vi "Read Sondenmodell.Zustandsgrössen.vi"(8 "error in (no error)":errorcluster, 11 "Sondenmodell in":refnum<class "Sondenmodell.lvclass">) -> (0 "error out":errorcluster, 2 "Sondenmodell.Zustandsgrössen":T1, 3 "Sondenmodell out":refnum<class "Sondenmodell.lvclass">)   [LabVIEW 2016, in "Sondenmodell.lvclass"]
uses:
  Sondenmodell.lvclass
  Sondenmodell.lvclass/Sondenmodell.ctl
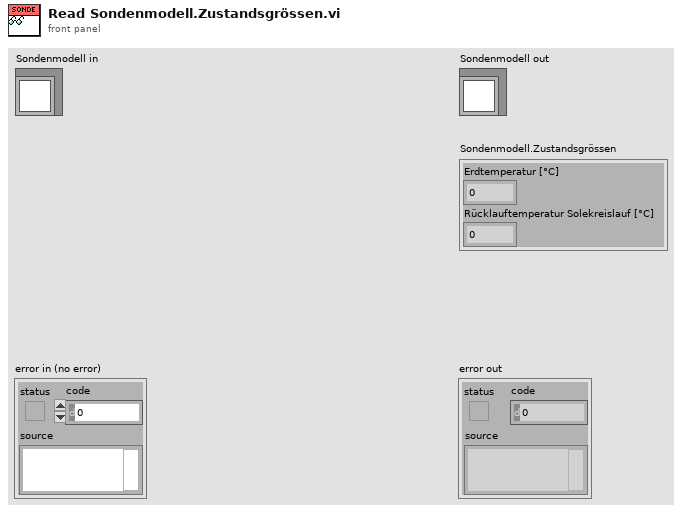
[diagram p1: front panel]
types:
  T1 = typedef "Sondenmodell.lvclass/Sondenmodell.Zustandsgrössen.ctl" = cluster{"Erdtemperatur [°C]":dbl, "Rücklauftemperatur Solekreislauf [°C]":dbl}
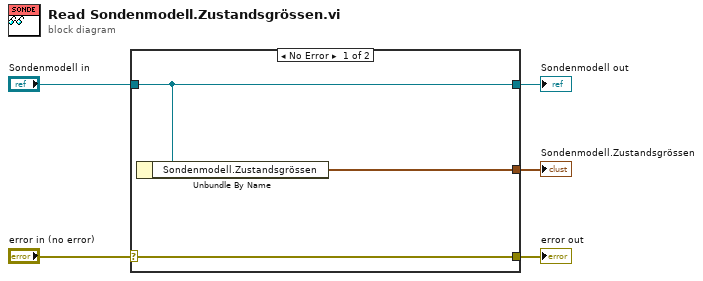
[diagram p0: block diagram]
diagram:
  n1 = case shown="No Error" "error in (no error)" {
    selector: "error in (no error)" -> [w8 w9]
    tunnel: [w8 w9] -> w4
    tunnel: [w7 w10] -> w2
    tunnel: "Sondenmodell in" -> [w7 w10]
    tunnel: [w6 _] -> w1
    frame No Error {
      n2 = Unbundle By Name(w7) -> ("Sondenmodell.Zustandsgrössen"=w6:T1)
    }
    frame Error {
    }
  }
  "error out" <- w4
  "Sondenmodell out" <- w2
  "Sondenmodell.Zustandsgrössen" <- w1
